vi "Examen_E3.vi"() -> ()   [LabVIEW 2024]
panel:
  out "Iteration":i32
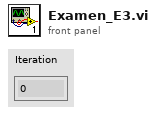
[diagram p1: front panel]
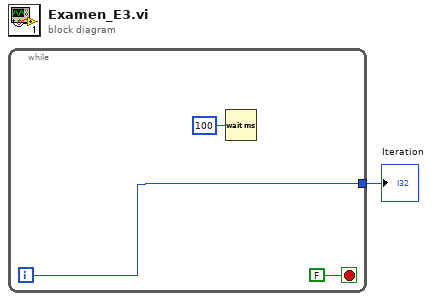
[diagram p0: block diagram]
diagram:
  n1 = while {
    tunnel: [w3] -> w1
    i -> [w3]
    stop <- FALSE stop-if-true
    n2 = Wait (ms)(milliseconds to wait=u32 100) -> ()  [unwired: 1 out]
  }
  "Iteration" <- w1
